vi "Power Accuracy Get Channel Data From Run Data.vi"(7 "Channel Name":string, 8 "error in (no error)":errorcluster, 10 "Run Waveforms":waveform(dbl)[](array[waveform]), 11 "File Information":T1) -> (0 "error out":errorcluster, 1 "Data Waveform":waveform(dbl), 3 "Found?":bool)   [LabVIEW 2011]
uses:
  server/TDMS/TDMS File.ctl
  server/TDMS/TDMS Run.ctl
  server/TDMS/TDMS Channel (Sxx).ctl
  server/database/Fields/Field Record.ctl
  server/database/Fields/Field DataTypes.ctl
  server/database/Fields/Field NextItem.ctl
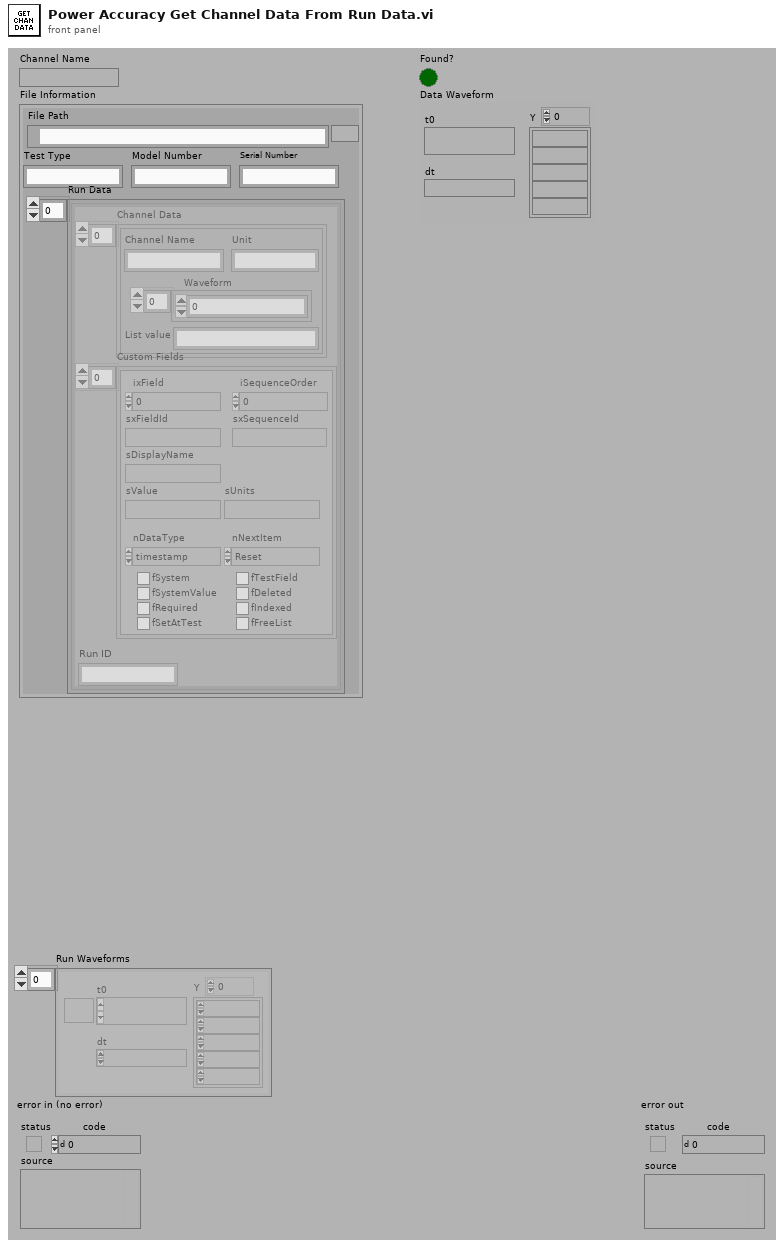
[diagram p1: front panel]
types:
  T1 = typedef "TDMS File.ctl" = cluster{"File Path":path, "Run Data":T2[], "Serial Number":string, "Model Number":string, "Test Type":string}
  T2 = typedef "TDMS Run.ctl" = cluster{"Channel Data":T3[], "Custom Fields":T4[], "Run ID":string}
  T3 = typedef "TDMS Channel (Sxx).ctl" = cluster{"Channel Name":string, "Waveform":dbl[], "Unit":string, "List value":string}
  T4 = typedef "Field Record.ctl" = cluster{"ixField":i32, "iSequenceOrder":i32, "sxFieldId":string, "sxSequenceId":string, "sDisplayName":string, "sValue":string, "sUnits":string, "nDataType":T5, "nNextItem":T6, "fSystem":bool, "fSystemValue":bool, "fRequired":bool, "fSetAtTest":bool, "fTestField":bool, "fDeleted":bool, "fIndexed":bool, "fFreeList":bool}
  T5 = typedef "Field DataTypes.ctl" = enum32{"text", "numeric", "list", "timestamp", "boolean"}
  T6 = typedef "Field NextItem.ctl" = enum32{"Reset", "Retain", "Auto-Increment"}
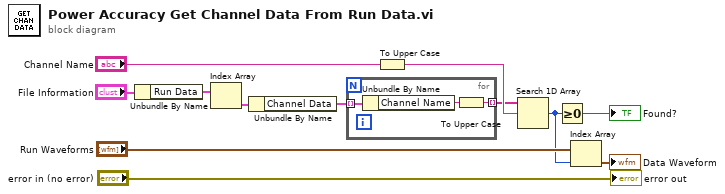
[diagram p0: block diagram]
diagram:
  n1 = Unbundle By Name("File Information") -> ("Run Data"=w10:T2[])
  n2 = Index Array(array=w10) -> (element=w11:T2)  [unwired: 1 in]
  n3 = Unbundle By Name(w11) -> ("Channel Data"=w8:T3[])
  n4 = for {
    tunnel: w8 -> [w15] mode=indexing
    tunnel: [w13] -> w6 mode=indexing
    n5 = Unbundle By Name(w15) -> ("Channel Name"=w14:string)
    n6 = To Upper Case(1:w14) -> (0:w13:string)
  }
  n7 = To Upper Case(1:"Channel Name") -> (0:w7:string)
  n8 = Search 1D Array(1D array=w6, element=w7) -> (index of element=w3:i32)  [unwired: 1 out]
  n9 = Greater Or Equal To 0?(x=w3) -> (x >= 0?=→"Found?":bool)
  n10 = Index Array(array="Run Waveforms", index=w3) -> (element=→"Data Waveform":waveform(dbl))
  "error out" <- "error in (no error)"
